vi "Update Count.vi"(0 "Guest Manager UI in":refnum<class "Guest Manager UI.lvclass">, 5 "Adult":bool, 7 "Increament":bool, 11 "error in (no error)":errorcluster) -> (4 "Guest Manager UI out":refnum<class "Guest Manager UI.lvclass">, 15 "error out":errorcluster)   [LabVIEW 2023, in "Guest Manager UI.lvlib" / "Guest Manager UI.lvclass"]
uses:
  Guest Manager UI.lvclass
  Guest Manager UI.lvclass/Guest Manager UI.ctl
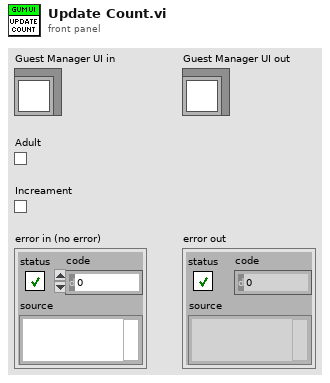
[diagram p1: front panel]
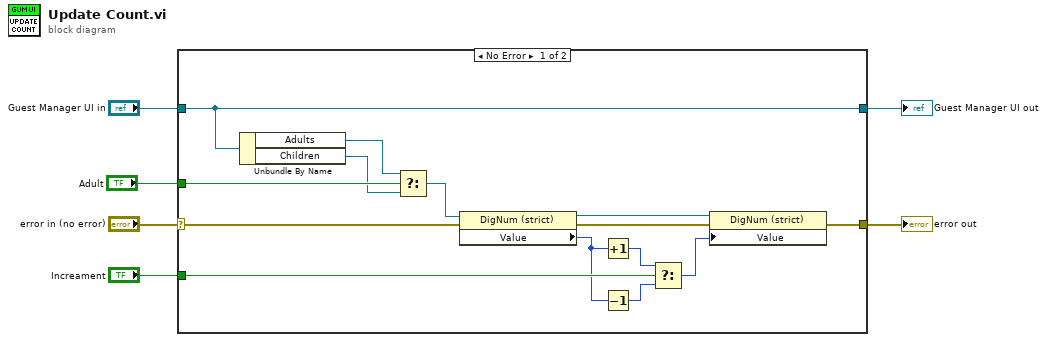
[diagram p0: block diagram]
diagram:
  n1 = case shown="No Error" "error in (no error)" {
    selector: "error in (no error)" -> [w20 w22]
    tunnel: [w17 w22] -> w5
    tunnel: [w19 w21] -> w3
    tunnel: "Guest Manager UI in" -> [w19 w21]
    tunnel: "Increament" -> [w15 _]
    tunnel: "Adult" -> [w9 _]
    frame No Error {
      n2 = Unbundle By Name(w19) -> ("Adults"=w10:refnum<vi>, "Children"=w8:refnum<vi>)
      n3 = Select(t=w10, s=w9, f=w8) -> (s? t:f=w7:refnum<vi>)
      n4 = property class="DigNum (strict)"(reference=w7, error in=w20) -> (reference out=w16:refnum<vi>, error out=w18:errorcluster, "Value"=w14:u32)
      n5 = Increment(x=w14) -> (x+1=w13:u32)
      n6 = Decrement(x=w14) -> (x-1=w12:u32)
      n7 = Select(t=w13, s=w15, f=w12) -> (s? t:f=w11:u32)
      n8 = property class="DigNum (strict)"(reference=w16, error in=w18, "Value"=w11) -> (error out=w17:errorcluster)  [unwired: 1 out]
    }
    frame Error {
    }
  }
  "error out" <- w5
  "Guest Manager UI out" <- w3
